vi "4.vi"(11 "文字列入力":string) -> (3 "文字列出力":string)   [LabVIEW 2019]
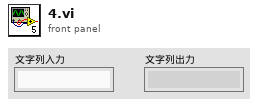
[diagram p1: front panel]
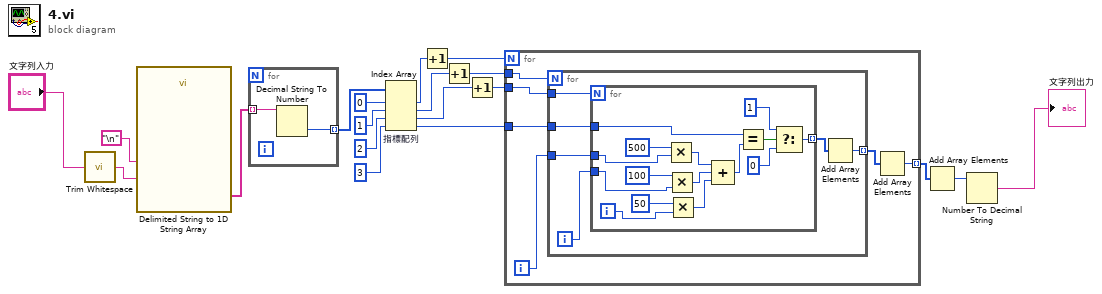
[diagram p0: block diagram]
diagram:
  n1 = call <vilib>:"Trim Whitespace.vi"("string"="文字列入力") -> ("trimmed string"=w6:string)  [unwired: 1 in]
  n2 = call <vilib>:"Delimited String to 1D String Array.vi"("delimiter"="\n", "delimited string"=w6) -> ("string array"=w9:string[])  [unwired: 9 in]
  n3 = for {
    tunnel: w9 -> [w21] mode=indexing
    tunnel: [w20] -> w10 mode=indexing
    n4 = Decimal String To Number(string=w21) -> (number=w20:i32)  [unwired: 2 in, 1 out]
  }
  n5 = Index Array "指標配列"(array=w10, index #1=0, index #2=1, index #3=2, index #4=3) -> (element #1=w14:i32, element #2=w16:i32, element #3=w18:i32, element #4=w11:i32)
  n6 = Increment(x=w14) -> (x+1=w15:i32)
  n7 = Increment(x=w16) -> (x+1=w17:i32)
  n8 = Increment(x=w18) -> (x+1=w19:i32)
  n9 = for {
    N: w15 -> [_]
    tunnel: w17 -> [w27]
    tunnel: w19 -> [w26]
    tunnel: w11 -> [w25]
    tunnel: [w22] -> w12 mode=indexing
    i -> [w24]
    n10 = for {
      N: w27 -> [_]
      tunnel: w26 -> [w33]
      tunnel: w25 -> [w32]
      tunnel: w24 -> [w31]
      tunnel: [w28] -> w23 mode=indexing
      i -> [w30]
      n11 = for {
        N: w33 -> [_]
        tunnel: w32 -> [w39]
        tunnel: w31 -> [w47]
        tunnel: w30 -> [w45]
        tunnel: [w35] -> w29 mode=indexing
        i -> [w43]
        n12 = Multiply(x=500, y=w47) -> (x*y=w42:i32)
        n13 = Multiply(x=100, y=w45) -> (x*y=w41:i32)
        n14 = Multiply(x=50, y=w43) -> (x*y=w40:i32)
        n15 = Compound Arithmetic op=ADD(w42, w41, w40) -> (w34:i32)
        n16 = Equal?(x=w39, y=w34) -> (x = y?=w38:bool)
        n17 = Select(t=1, s=w38, f=0) -> (s? t:f=w35:i32)
      }
      n18 = Add Array Elements(numeric array=w29) -> (sum=w28:i32)
    }
    n19 = Add Array Elements(numeric array=w23) -> (sum=w22:i32)
  }
  n20 = Add Array Elements(numeric array=w12) -> (sum=w13:i32)
  n21 = Number To Decimal String(number=w13) -> (decimal integer string=→"文字列出力":string)  [unwired: 1 in]
